vi "CreateTopic.vi"(8 "error in (no error)":errorcluster, 9 "1:M":bool, 10 "Topic Name":string, 11 "Message Broker in":refnum<class "Message Broker.lvclass">) -> (0 "error out":errorcluster, 2 "Locked?":bool, 3 "Message Broker out":refnum<class "Message Broker.lvclass">, 5 "Transport":refnum<class "Message Transport Queue.lvclass">)   [LabVIEW 2016, in "Stream Mediator.lvlib" / "Message Broker.lvclass"]
doc: "--\nCopyright © 2017 Composed SystemsI All rights reserved.\n\nAuthor: Jon McBee <jon.mcbee@composed.io>\n\nThis library is provided \"AS IS\" ,WITHOUT WARRANTIES OR\nCONDITIONS OF ANY KIND, either express or implied.\n\nComposed Systems -- composed.io\n\nStream 0.0.1.1\nJon McBee - Composed Systems\nCopyright (c) 2017, Composed Systems"
uses:
  <userlib>/Composed Systems/Stream/Mediator/Classes/Message Broker/Message Broker.lvclass
  <userlib>/Composed Systems/Stream/Mediator/Classes/Message Transport Queue/Message Transport Queue.lvclass
  <userlib>/Composed Systems/Stream/Mediator/Classes/Message Broker/Message Broker.lvclass/Message Broker.ctl
  <userlib>/Composed Systems/Stream/Mediator/Classes/Topic Actor Descriptor/Topic Actor Descriptor.lvclass
  <userlib>/Composed Systems/Stream/Mediator/Classes/Topic Actor/Topic Actor.lvclass
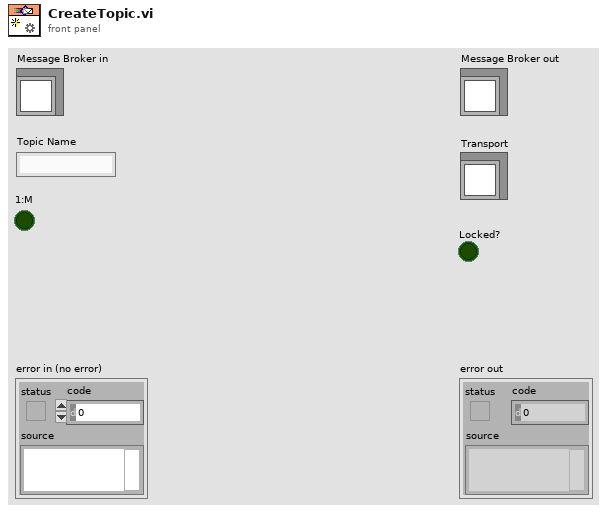
[diagram p1: front panel]
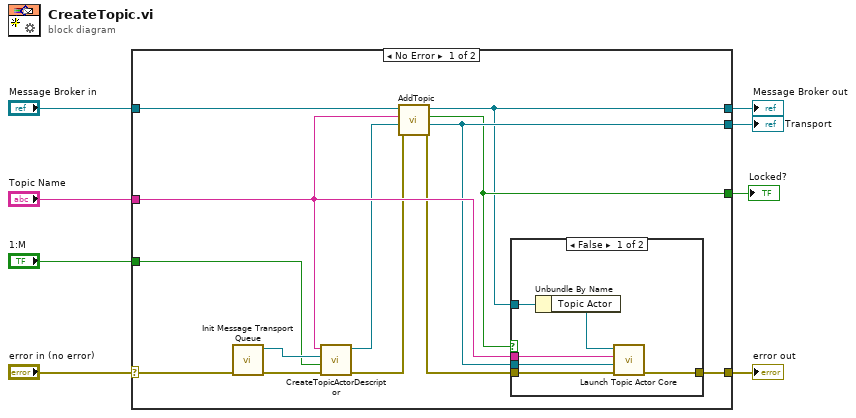
[diagram p0: block diagram]
diagram:
  n1 = case shown="No Error" "error in (no error)" {
    selector: "error in (no error)" -> [w21 w30]
    tunnel: [w15 w30] -> w7
    tunnel: [w9 w29] -> w5
    tunnel: "Message Broker in" -> [w17 w29]
    tunnel: "Topic Name" -> [w16 _]
    tunnel: "1:M" -> [w18 _]
    tunnel: [w11 _] -> w2
    tunnel: [w10 _] -> w1
    frame No Error {
      n2 = call <userlib>:"Init Message Transport Queue.vi"("error in (no error)"=w21) -> ("error out"=w19:errorcluster, "Message Transport Queue out"=w20:refnum<class "Message Transport Queue.lvclass">)  [unwired: 9 in]
      n3 = call <userlib>:"CreateTopicActorDescriptor.vi"("error in (no error)"=w19, "1:M"=w18, "Transport"=w20, "Name"=w16) -> ("error out"=w13:errorcluster, "Topic Actor Descriptor out"=w14:refnum<class "Topic Actor Descriptor.lvclass">)  [unwired: 6 in]
      n4 = call <userlib>:"AddTopic.vi"("error in (no error)"=w13, "Topic Actor Descriptor"=w14, "Topic Name"=w16, "Message Broker in"=w17) -> ("error out"=w12:errorcluster, "Transport"=w11:refnum<class "Message Transport Queue.lvclass">, "Locked?"=w10:bool, "Message Broker out"=w9:refnum<class "Message Broker.lvclass">)  [unwired: 4 in]
      n5 = case shown="False" w10 {
        tunnel: w16 -> [w27 _]
        tunnel: [w26 w28] -> w15
        tunnel: w12 -> [w25 w28]
        tunnel: w11 -> [w24 _]
        tunnel: w9 -> [w23 _]
        frame False {
          n6 = Unbundle By Name(w23) -> ("Topic Actor"=w22:refnum<class "Topic Actor.lvclass">)
          n7 = call <userlib>:"Launch Topic Actor Core.vi"("error in (no error)"=w25, "Inbox"=w24, "Topic Name"=w27, "Topic Actor in"=w22) -> ("error out"=w26:errorcluster)  [unwired: 7 in]
        }
        frame True {
        }
      }
    }
    frame Error {
    }
  }
  "error out" <- w7
  "Message Broker out" <- w5
  "Transport" <- w2
  "Locked?" <- w1
